vi "Add Descendent Items.vi"(8 "error in (no error)":errorcluster, 9 "Order":i32, 11 "Descendents Refs":refnum<vi>[](array[refnum])) -> (0 "error out":errorcluster, 3 "Items":refnum<class "Item.lvclass">[](array[class]))   [LabVIEW 2020, in "VI Properties Editor.lvlib"]
doc: "Initializes class data for the items identified by <B>Descendents Refs</B>, taking into account the <B>Order</B> in which they appear in the Project Explorer window."
uses:
  VI Properties Editor.lvlib
  Classes/Item/Item.lvclass
  Classes/Support/Item Type.ctl
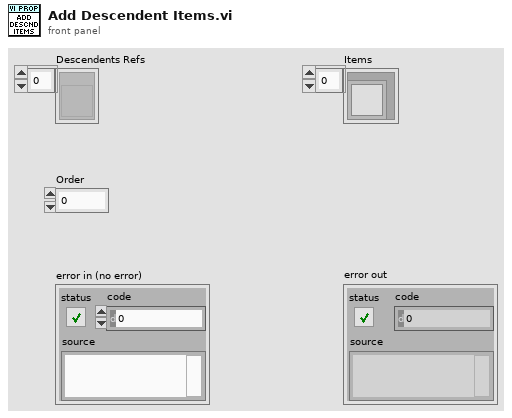
[diagram p1: front panel]
types:
  T1 = typedef "imagedata.ctl" = cluster{"image type":i32, "image depth":i32, "image":u8[], "mask":u8[], "colors":u32[], "Rectangle":cluster{"left":i16, "top":i16, "right":i16, "bottom":i16}}
  T2 = cluster{"Private":T1, "Protected":T1, "Community":T1}
  T3 = typedef "VI Properties Editor.lvlib/Item Type.ctl" = enum16{"Generic", "VI"}
  T4 = enum32{"invalid scope", "public", "private", "protected", "community"}
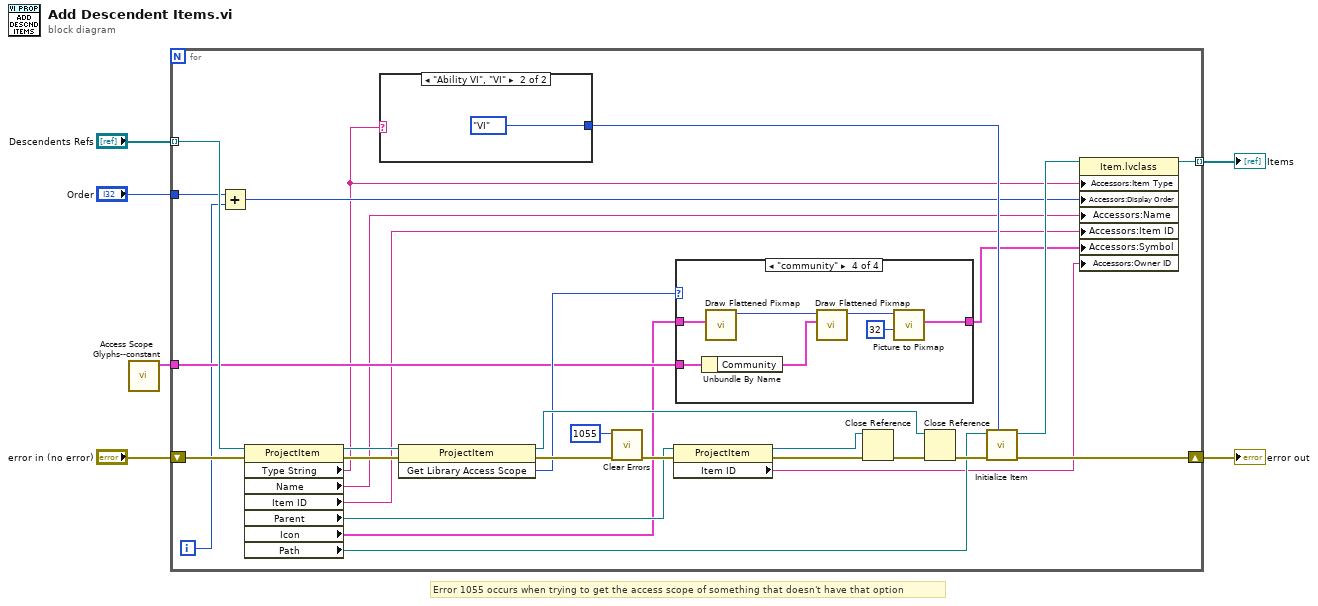
[diagram p0: block diagram]
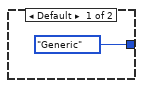
[diagram p2: hidden frame]
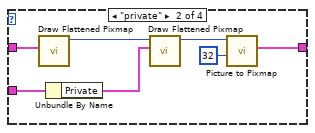
[diagram p4: hidden frame]
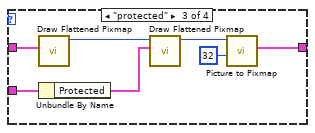
[diagram p5: hidden frame]
diagram:
  # "Error 1055 occurs when trying to get the access scope of something that doesn't have that option"
  n1 = call "Access Scope Glyphs--constant.vi"() -> ("Access Scope Glyphs"=w2:T2)  [unwired: 11 in]
  n2 = for {
    shift-right: [w30] -> w5
    shift-left: "error in (no error)" -> [w34]
    tunnel: "Descendents Refs" -> [w26] mode=indexing
    tunnel: w2 -> [w21]
    tunnel: "Order" -> [w20]
    tunnel: [w13] -> w1 mode=indexing
    i -> [w19]
    n3 = Add(x=w20, y=w19) -> (x+y=w12:i32)
    n4 = property class="ProjectItem"(reference=w26, error in=w34) -> (reference out=w27:refnum<vi>, error out=w33:errorcluster, "Type String"=w11:string, "Name"=w10:string, "Item ID"=w8:string, "Parent"=w25:refnum<vi>, "Icon"=w17:T1, "Path"=w15:path)
    n5 = case shown="\"Ability VI\", \"VI\"" w11 {
      tunnel: [Item_Type."Generic" ("Item Type") Item_Type."VI" ("Item Type")] -> w16
      frame Default {
      }
      frame "Ability VI", "VI" {
      }
    }
    n6 = invoke class="ProjectItem" method="Get Library Access Scope"(reference=w27, error in=w33) -> (reference out=w23:refnum<vi>, error out=w32:errorcluster, "Get Library Access Scope"=w22:T4)  [unwired: 1 in]
    n7 = call <vilib>:"Clear Errors.vi"("error in (no error)"=w32, "specific error code to clear (0: all)"=1055) -> ("error out"=w35:errorcluster)  [unwired: 4 in, 1 out]
    n8 = property class="ProjectItem"(reference=w25, error in=w35) -> (reference out=w24:refnum<vi>, error out=w31:errorcluster, "Item ID"=w9:string)
    n9 = case shown="\"community\"" w22 {
      tunnel: w21 -> [_ w40 w47 w54]
      tunnel: w17 -> [w38 w45 w52 w59]
      tunnel: [w38 w42 w49 w56] -> w7
      frame "invalid scope", "public" {
      }
      frame "private" {
        n10 = call <vilib>:"Draw Flattened Pixmap.vi"("image data"=w45) -> ("new picture"=w44:picture)  [unwired: 8 in]
        n11 = Unbundle By Name(w40) -> ("Private"=w39:T1)
        n12 = call <vilib>:"Draw Flattened Pixmap.vi"("image data"=w39, "picture"=w44) -> ("new picture"=w43:picture)  [unwired: 7 in]
        n13 = call <vilib>:"Picture to Pixmap.vi"("depth"=32, "picture"=w43) -> ("image data"=w42:T1)  [unwired: 8 in, 1 out]
      }
      frame "protected" {
        n14 = call <vilib>:"Draw Flattened Pixmap.vi"("image data"=w52) -> ("new picture"=w51:picture)  [unwired: 8 in]
        n15 = Unbundle By Name(w47) -> ("Protected"=w46:T1)
        n16 = call <vilib>:"Draw Flattened Pixmap.vi"("image data"=w46, "picture"=w51) -> ("new picture"=w50:picture)  [unwired: 7 in]
        n17 = call <vilib>:"Picture to Pixmap.vi"("depth"=32, "picture"=w50) -> ("image data"=w49:T1)  [unwired: 8 in, 1 out]
      }
      frame "community" {
        n18 = Unbundle By Name(w54) -> ("Community"=w53:T1)
        n19 = call <vilib>:"Draw Flattened Pixmap.vi"("image data"=w59) -> ("new picture"=w58:picture)  [unwired: 8 in]
        n20 = call <vilib>:"Draw Flattened Pixmap.vi"("image data"=w53, "picture"=w58) -> ("new picture"=w57:picture)  [unwired: 7 in]
        n21 = call <vilib>:"Picture to Pixmap.vi"("depth"=32, "picture"=w57) -> ("image data"=w56:T1)  [unwired: 8 in, 1 out]
      }
    }
    n22 = Close Reference(reference=w24, error in (no error)=w31) -> (error out=w29:errorcluster)
    n23 = Close Reference(reference=w23, error in (no error)=w29) -> (error out=w28:errorcluster)
    n24 = call "Initialize Item.vi"("Item Type"=w16, "error in (no error)"=w28, "Path"=w15) -> ("error out"=w30:errorcluster, "Item"=w14:refnum<class "Item.lvclass">)  [unwired: 7 in]
    n25 = property class="Item.lvclass"(reference=w14, "Accessors:Item Type"=w11, "Accessors:Display Order"=w12, "Accessors:Name"=w10, "Accessors:Item ID"=w8, "Accessors:Symbol"=w7, "Accessors:Owner ID"=w9) -> (reference out=w13:refnum<class "Item.lvclass">)  [unwired: 1 in, 1 out]
  }
  "error out" <- w5
  "Items" <- w1
